vi "FTW-Inbox-Construct.vi"(5 "Primary Inbox Address":string, 7 "Inbox Configuration":string, 11 "error in":errorcluster) -> (4 "FTW Router":refnum<data-value>, 6 "Resolved Primary Inbox Address":string, 8 "Incoming Request":refnum<event-registration>, 15 "error out":errorcluster)   [LabVIEW 2014]
uses:
  core/FTW-Inbox-Core-CallbackParameters.ctl
  core/FTW-Inbox-Core-RoutingRule.ctl
  core/FTW-Inbox-Core-Type.ctl
  json/core/FTW-JSON-Core-Structure.ctl
panel:
  # "Inputs"
  # "Outputs"
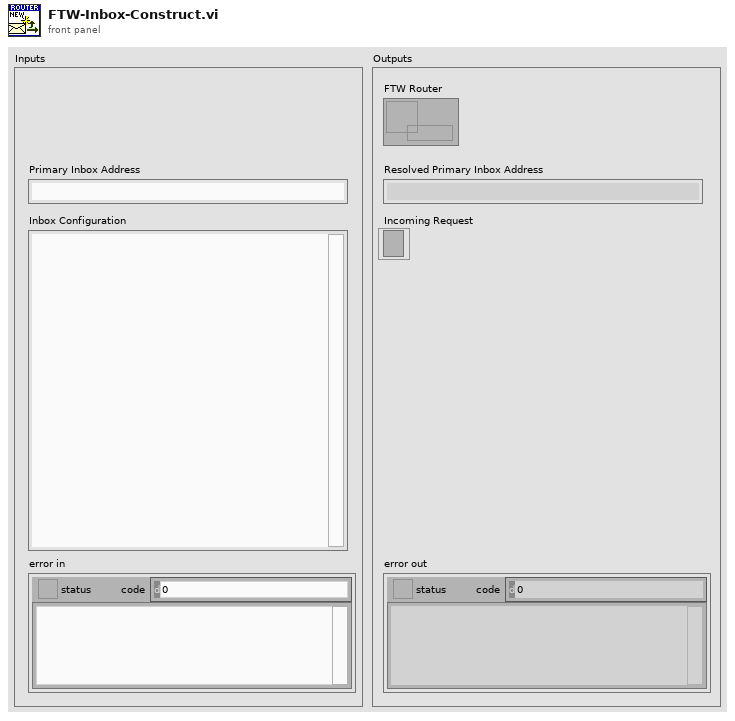
[diagram p1: front panel]
types:
  T1 = typedef "FTW-Inbox-Core-RoutingRule.ctl" = cluster{"Pattern":string, "BusyTimeout":i32, "SendTimeout":i32, "Accept":bool, "Reject":bool, "ReplyWithIdentity":bool, "ReplyWithStats":bool, "ReplyWithTimestamp":bool, "ReplyWithRelativeTimer":bool, "AutoReply":bool}
  T2 = typedef "FTW-Inbox-Core-CallbackParameters.ctl" = cluster{"MessageNotifier":refnum<user-event>, "MessagePipe":refnum<queue>, "Routing Rules":T1[], "Actor Identity":string, "Statistics":refnum<data-value>}
  T3 = typedef "FTW-Inbox-Core-Type.ctl" = cluster{"Socket":i64, "MessageNotifier":refnum<user-event>, "Message Broker":refnum<user-event>}
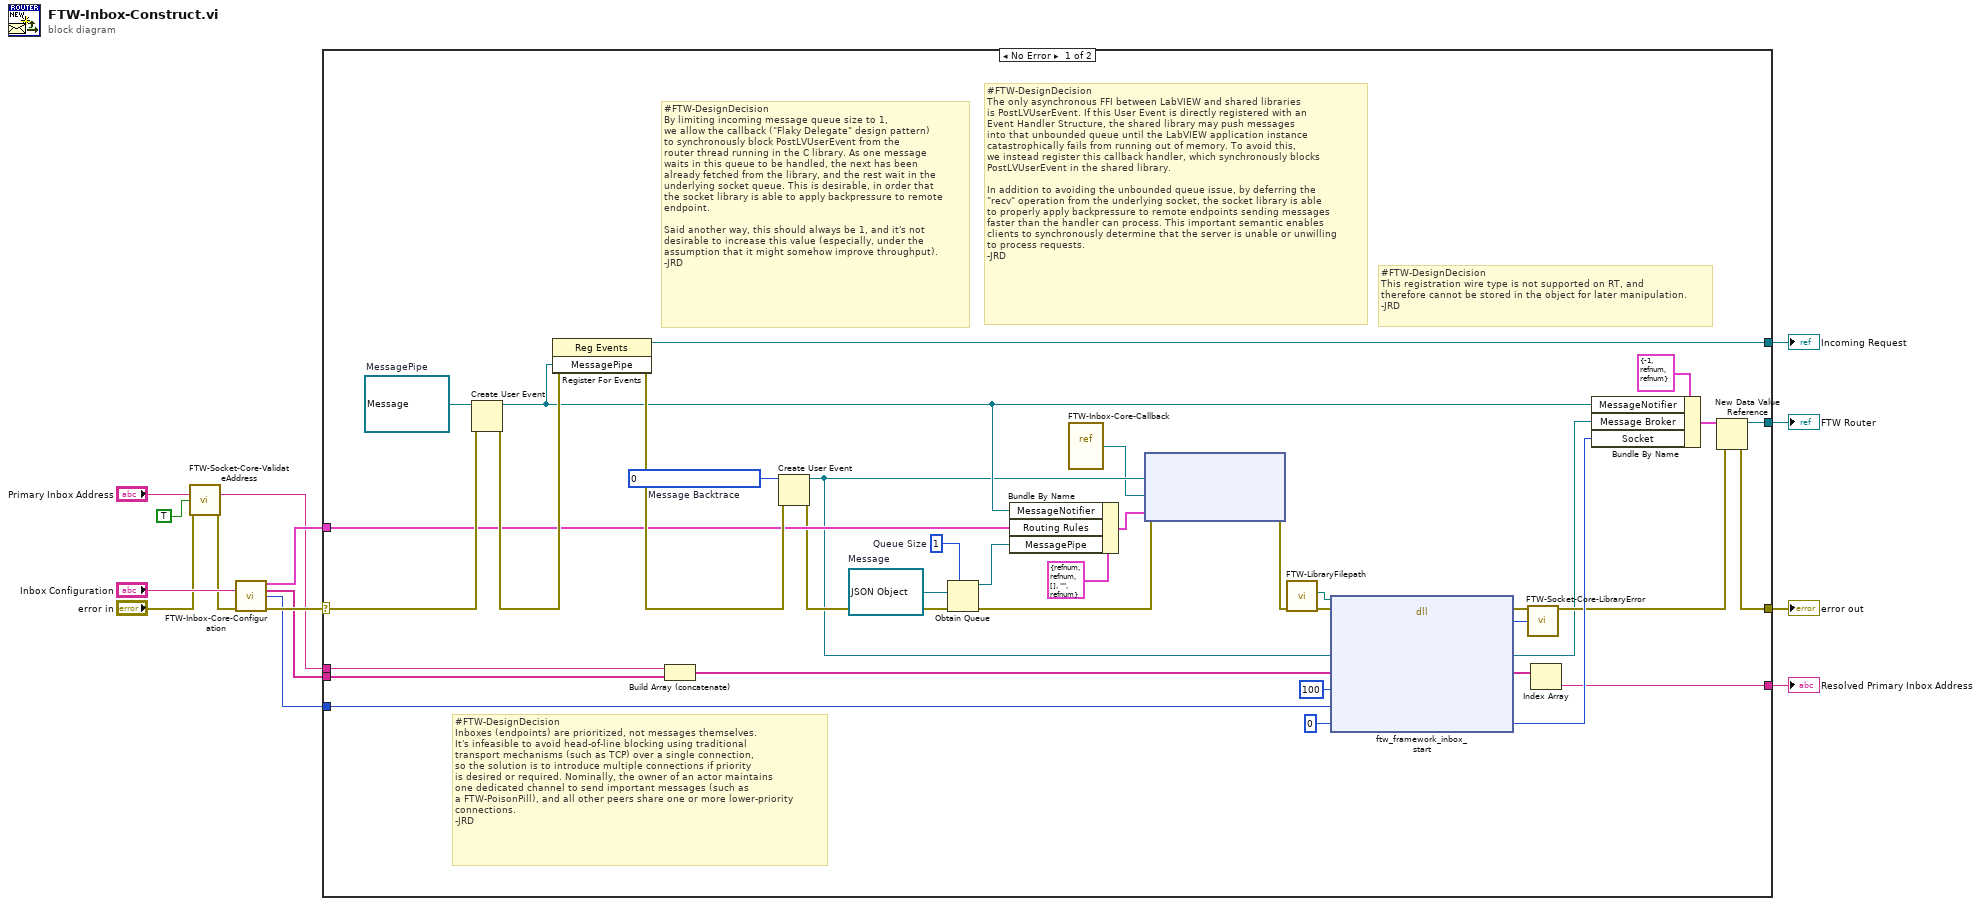
[diagram p0: block diagram]
diagram:
  n1 = call "FTW-Socket-Core-ValidateAddress.vi"("Address"="Primary Inbox Address", "Allow wildcard replacement?"=TRUE, "error in"="error in") -> ("Sanitized Address"=w3:string, "error out"=w4:errorcluster)  [unwired: 10 in, 1 out]
  n2 = call "FTW-Inbox-Core-Configuration.vi"("Inbox Configuration"="Inbox Configuration", "error in"=w4) -> ("Message Routing Rules"=w8:T1[], "Additional Endpoint Addresses"=w2:string[], "Receive Message Size Limit"=w1:i32, "error out"=w10:errorcluster)  [unwired: 9 in, 1 out]
  n3 = case shown="No Error" w10 {
    selector: w10 -> [w46 w52]
    tunnel: [w38 _] -> w14
    tunnel: [w36 w52] -> w13
    tunnel: [w47 _] -> w11
    tunnel: w3 -> [w26 _]
    tunnel: [w22 _] -> w12
    tunnel: w1 -> [w34 _]
    tunnel: w8 -> [w32 _]
    tunnel: w2 -> [w24 _]
    frame No Error {
      w19 = i64 0  # Message Backtrace
      w27 = refnum<data-value> refnum  # Message
      w30 = 1  # Queue Size
      w35 = refnum<queue> refnum  # MessagePipe
      # "#FTW-DesignDecision\nThe only asynchronous FFI between LabVIEW and shared libraries\nis PostLVUserEvent. If this User Event is directly registered with an\nEvent Handler Structure, the shared library may push messages\ninto that unbounded queue until the LabVIEW application instance\ncatastrophically fails from running out of memory. To avoid this,\nwe instead register this callback handler, which synchronously blocks\nPostLVUserEvent in the shared library.\n\nIn addition to avoiding the unbounded queue issue, by deferring the\n\"recv\" operation from the underlying socket, the socket library is able\nto properly apply backpressure to remote endpoints sending messages\nfaster than the handler can process. This important semantic enables\nclients to synchronously determine that the server is unable or unwilling\nto process requests.\n-JRD"
      # "#FTW-DesignDecision\nBy limiting incoming message queue size to 1,\nwe allow the callback (\"Flaky Delegate\" design pattern)\nto synchronously block PostLVUserEvent from the\nrouter thread running in the C library. As one message\nwaits in this queue to be handled, the next has been\nalready fetched from the library, and the rest wait in the\nunderlying socket queue. This is desirable, in order that\nthe socket library is able to apply backpressure to remote\nendpoint.\n\nSaid another way, this should always be 1, and it's not\ndesirable to increase this value (especially, under the\nassumption that it might somehow improve throughput).\n-JRD"
      # "#FTW-DesignDecision\nThis registration wire type is not supported on RT, and\ntherefore cannot be stored in the object for later manipulation.\n-JRD"
      # "#FTW-DesignDecision\nInboxes (endpoints) are prioritized, not messages themselves.\nIt's infeasible to avoid head-of-line blocking using traditional\ntransport mechanisms (such as TCP) over a single connection,\nso the solution is to introduce multiple connections if priority\nis desired or required. Nominally, the owner of an actor maintains\none dedicated channel to send important messages (such as\na FTW-PoisonPill), and all other peers share one or more lower-priority\nconnections.\n-JRD"
      n4 = Create User Event(user event datatype=w35, error in=w46) -> (user event=w20:refnum<user-event>, error out=w45:errorcluster)
      n5 = register-events(error in=w45, w20) -> (reference out=w47:refnum<event-registration>, error out=w43:errorcluster)  [unwired: 1 in]
      n6 = Build Array (concatenate)(w26, w24) -> (w25:string[])
      n7 = Create User Event(user event datatype=w19, error in=w43) -> (user event=w18:refnum<user-event>, error out=w28:errorcluster)
      n8 = Obtain Queue(max queue size (-1, unlimited)=w30, element data type=w27, error in (no error)=w28) -> (queue out=w15:refnum<queue>, error out=w29:errorcluster)  [unwired: 2 in, 1 out]
      n9 = Bundle By Name(cluster=T2 {"MessageNotifier"=refnum, "MessagePipe"=refnum, "Routing Rules"=[], "Actor Identity"="", "Statistics"=refnum} ("Callback Parameters"), "MessageNotifier"=w20, "Routing Rules"=w32, "MessagePipe"=w15) -> (w17:T2)
      n10 = vi-ref "FTW-Inbox-Core-Callback.vi"() -> (w16:refnum<vi>)
      n11 = node(w29, w18, w16, w17) -> (w44:errorcluster)  [unwired: 1 in, 1 out]
      n12 = call "FTW-LibraryFilepath.vi"("error in"=w44) -> ("error out"=w50:errorcluster, "Library Filepath"=w51:path)  [unwired: 8 in, 1 out]
      n13 = dll-call lib="?" fn="ftw_framework_inbox_start"(path in=w51, error in=w50, "Incoming Message \"Notifier\""=w18, "Addresses"=w25, "Linger (msec)"=100, "Max Recv Size (bytes)"=w34, "Socket Handle"=i64 0) -> (error out=w49:errorcluster, "Return Value"=w48:i64, "Incoming Message \"Notifier\""=w21:refnum<user-event>, "Addresses"=w23:string[], "Socket Handle"=w41:i64)  [unwired: 5 in, 1 out]
      n14 = call "FTW-Socket-Core-LibraryError.vi"("error in"=w49, "Return Value"=w48) -> ("error out"=w37:errorcluster)  [unwired: 13 in]
      n15 = Index Array(array=w23) -> (element=w22:string)  [unwired: 1 in]
      n16 = Bundle By Name(cluster=T3 {"Socket"=-1, "MessageNotifier"=refnum, "Message Broker"=refnum} ("FTW Router"), "MessageNotifier"=w20, "Message Broker"=w21, "Socket"=w41) -> (w39:T3)
      n17 = New Data Value Reference(data value=w39, error in=w37) -> (data value reference=w38:refnum<data-value>, error out=w36:errorcluster)
    }
    frame Error {
    }
  }
  "error out" <- w13
  "FTW Router" <- w14
  "Resolved Primary Inbox Address" <- w12
  "Incoming Request" <- w11
